vi "CSU22 Send Command.vi"(0 "VISA Ref":refnum<visa-resource-name>, 2 "Wait for Reply (T)":bool=TRUE, 7 "Command":string, 11 "Error In":errorcluster) -> (4 "VISA Ref Dup":refnum<visa-resource-name>, 8 "Reply":string, 10 "Success?":bool, 15 "Error Out":errorcluster)   [LabVIEW 2020]
uses:
  <vilib>/Utility/error.llb/whitespace.ctl
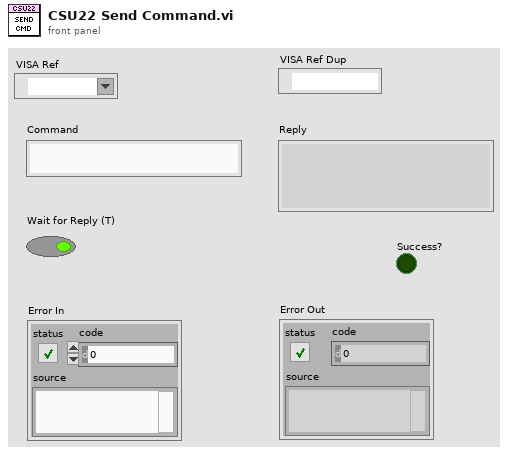
[diagram p1: front panel]
types:
  T1 = typedef "whitespace.ctl" = u16
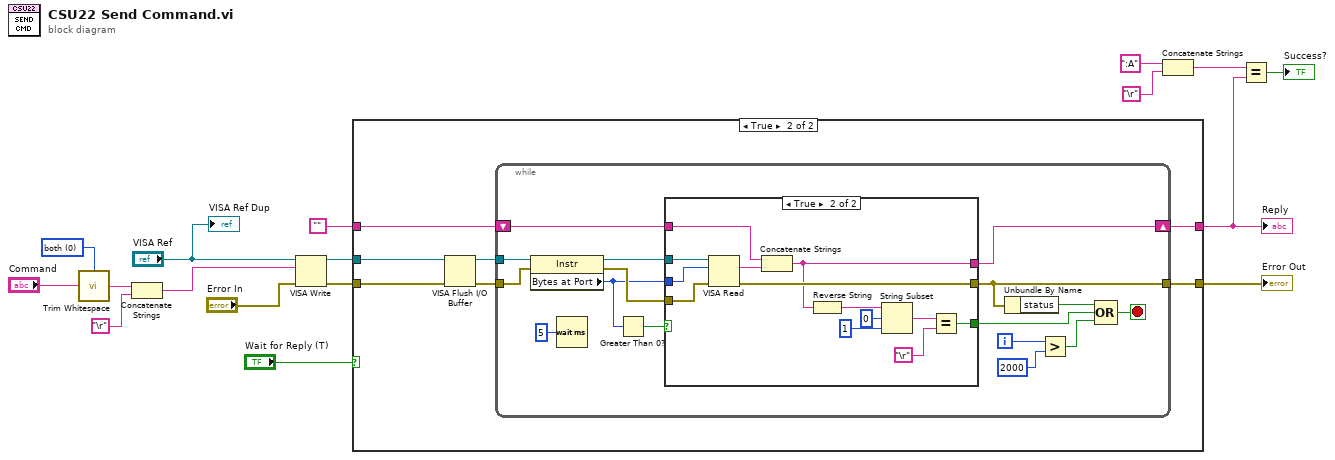
[diagram p0: block diagram]
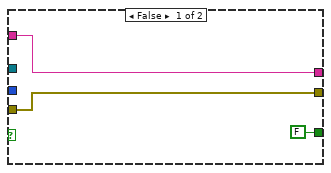
[diagram p3: hidden frame]
diagram:
  w16 = T1 0 items=["both", "start of string", "end of string"] ("location (both)")
  n1 = call <vilib>:"Trim Whitespace.vi"("string"="Command", "location (both)"=w16) -> ("trimmed string"=w15:string)
  n2 = Concatenate Strings(w15, "\r") -> (w13:string)
  n3 = VISA Write(VISA resource name="VISA Ref", write buffer=w13, error in (no error)="Error In") -> (VISA resource name out=w12:refnum<visa-resource-name>, error out=w11:errorcluster)  [unwired: 1 out]
  n4 = case shown="True" "Wait for Reply (T)" {
    tunnel: w12 -> [_ w23]
    tunnel: w11 -> [w19 w21]
    tunnel: "" -> [w18 w26]
    tunnel: [w18 w25] -> w5
    tunnel: [w19 w24] -> w7
    frame False {
    }
    frame True {
      n5 = VISA Flush I/O Buffer(VISA resource name=w23, error in (no error)=w21) -> (VISA resource name out=w22:refnum<visa-resource-name>, error out=w20:errorcluster)  [unwired: 1 in]
      n6 = while {
        tunnel: w22 -> [w42]
        tunnel: w20 -> [w41]
        shift-right: [w30] -> w25
        shift-left: w26 -> [w31]
        tunnel: [w27] -> w24
        i -> [w40]
        stop <- w37 stop-if-true
        n7 = property class="Instr"(reference=w42, error in=w41) -> (reference out=w33:refnum<visa-resource-name>, error out=w34:errorcluster, "Bytes at Port"=w32:u32)
        n8 = Wait (ms)(milliseconds to wait=u32 5) -> ()  [unwired: 1 out]
        n9 = Greater Than 0?(x=w32) -> (x > 0?=w35:bool)
        n10 = case shown="True" w35 {
          tunnel: w34 -> [w44 w57]
          tunnel: w33 -> [_ w58]
          tunnel: w32 -> [_ w56]
          tunnel: w31 -> [w45 w55]
          tunnel: [w45 w52] -> w30
          tunnel: [w44 w53] -> w27
          tunnel: [FALSE w46] -> w28
          frame False {
          }
          frame True {
            n11 = VISA Read(VISA resource name=w58, byte count=w56, error in (no error)=w57) -> (read buffer=w54:string, error out=w53:errorcluster)  [unwired: 2 out]
            n12 = Concatenate Strings(w55, w54) -> (w52:string)
            n13 = Reverse String(1:w52) -> (0:w51:string)
            n14 = String Subset(string=w51, offset (0)=0, length (rest)=1 ("length (rest)")) -> (substring=w48:string)
            n15 = Equal?(x=w48, y="\r") -> (x = y?=w46:bool)
          }
        }
        n16 = Unbundle By Name(w27) -> ("status"=w29:bool)
        n17 = Greater?(x=w40, y=2000) -> (0:w38:bool)
        n18 = Compound Arithmetic op=OR(w29, w28, w38) -> (w37:bool)
      }
    }
  }
  "Reply" <- w5
  "Error Out" <- w7
  n19 = Concatenate Strings(":A" ("string"), "\r") -> (w2:string)
  n20 = Equal?(x=w2, y=w5) -> (x = y?=→"Success?":bool)
  "VISA Ref Dup" <- "VISA Ref"
